vi "GalvoPointScanSet.vi"(8 "error in (no error)":errorcluster, 9 "Cursor Position (V)":cluster{"Cursor X":dbl, "Cursor Y":dbl}, 10 "task in":refnum<k21>, 11 "Microscope in":refnum<class "Microscope.lvclass">) -> (0 "error out":errorcluster, 2 "task out":refnum<k21>, 3 "Microscope out":refnum<class "Microscope.lvclass">)   [LabVIEW 2012, in "Microscope.lvclass"]
uses:
  classes/Microscope.lvclass
  classes/Microscope.lvclass/Microscope.ctl
  <vilib>/DAQmx/write.llb/DAQmx Write (Analog 2D DBL NChan NSamp).vi
  <vilib>/DAQmx/miscellaneous.llb/DAQmx Fill In Error Info.vi
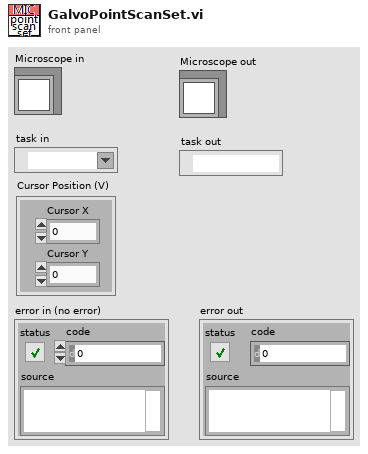
[diagram p1: front panel]
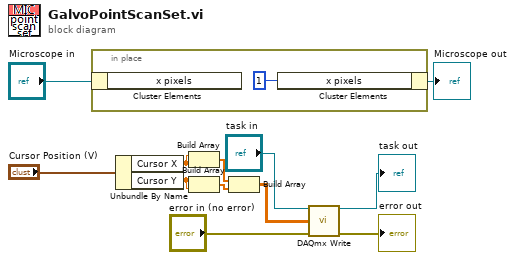
[diagram p0: block diagram]
diagram:
  n1 = in-place {
    n2 = in-place-cluster #1("Microscope in") -> ()  [unwired: 1 out]
    n3 = in-place-cluster #1("x pixels"=1 ("Scan Parameters.x pixels")) -> (→"Microscope out":refnum<class "Microscope.lvclass">)
  }
  n4 = Unbundle By Name("Cursor Position (V)") -> ("Cursor X"=w2:dbl, "Cursor Y"=w1:dbl)
  n5 = Build Array(w2, w2) -> (w8:dbl[])
  n6 = Build Array(w1, w1) -> (w9:dbl[])
  n7 = Build Array(w8, w9) -> (w10:dbl[][])
  n8 = call-poly <vilib>:"DAQmx Write.vi"("task/channels in"="task in", "data"=w10, "error in"="error in (no error)") -> ("task out"=→"task out":refnum<k21>, "error out"=→"error out":errorcluster)  [unwired: 10 in, 1 out]
